vi "Control commands to FPGA.vi"(0 "Refnum in":refnum<k20>, 1 "error in (no error)":errorcluster, 2 "LQR direction":bool, 3 "Duty cycle (Only used for LQR)":dbl, 4 "Controller output":dbl, 6 "Reset steering angle":bool, 8 "Reset steering\nposition controller":bool) -> (14 "Refnum out":refnum<k20>, 15 "error out":errorcluster, 19 "Log?":dbl)   [LabVIEW 2016]
uses:
  <vilib>/Utility/error.llb/Error Cluster From Error Code.vi
  <vilib>/rvi/errors/niLvFpgaAdjustHostInterfaceError.vi
  <vilib>/rvi/interface/nirviReadWriteControl/nirviReadWriteControl.xnode
  NiFpgaLv.dll
  <vilib>/rvi/interface/Simulation/niFpgaSimulationCallBeginRW.vi
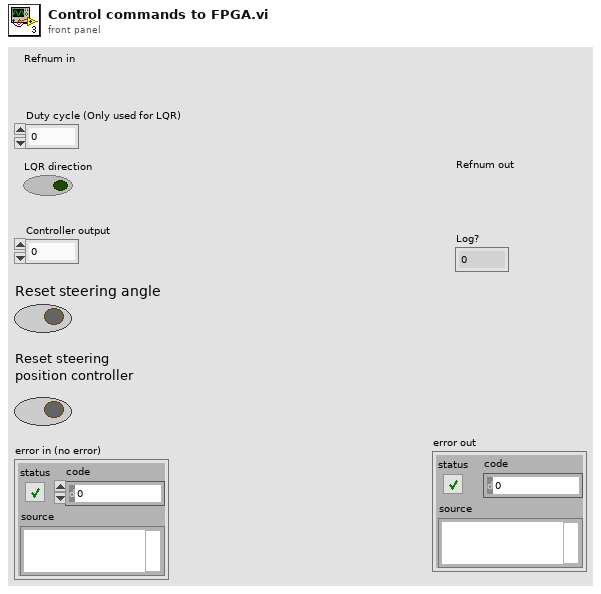
[diagram p1: front panel]
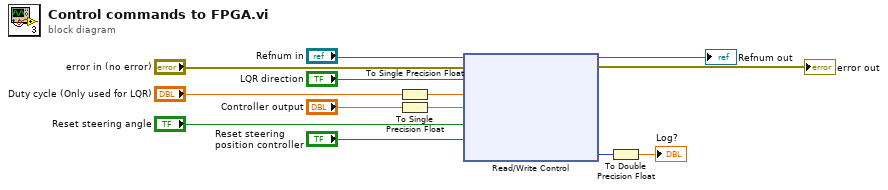
[diagram p0: block diagram]
diagram:
  n1 = To Single Precision Float(number="Duty cycle (Only used for LQR)") -> (single precision float=w9:sgl)
  n2 = To Single Precision Float(number="Controller output") -> (single precision float=w11:sgl)
  n3 = xnode "Read/Write Control"("FPGA VI Reference In"="Refnum in", "error in"="error in (no error)", "LQR Direction"="LQR direction", "LQR Duty Cycle"=w9, "Desired steering angle"=w11, "Reset counter"="Reset steering angle", "Steering PID reset?"="Reset steering\nposition controller") -> ("FPGA VI Reference Out"=→"Refnum out":refnum<k20>, "error out"=→"error out":errorcluster, "Channel 7 position"=w7:u8)
  n4 = To Double Precision Float(number=w7) -> (double precision float=→"Log?":dbl)
